vi "SetOpenWindow.vi"(8 "error in (no error)":errorcluster, 10 "Open Window":bool, 11 "object in":refnum<class "Vi_Button.lvclass">) -> (0 "error out":errorcluster, 3 "object out":refnum<class "Vi_Button.lvclass">)   [LabVIEW 2012, in "Vi_Button.lvclass"]
uses:
  Vi_Button.lvclass
  Vi_Button.lvclass/Vi_Button.ctl
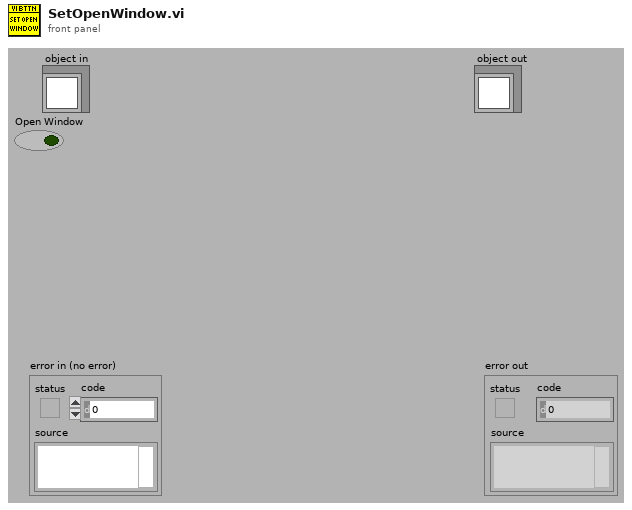
[diagram p1: front panel]
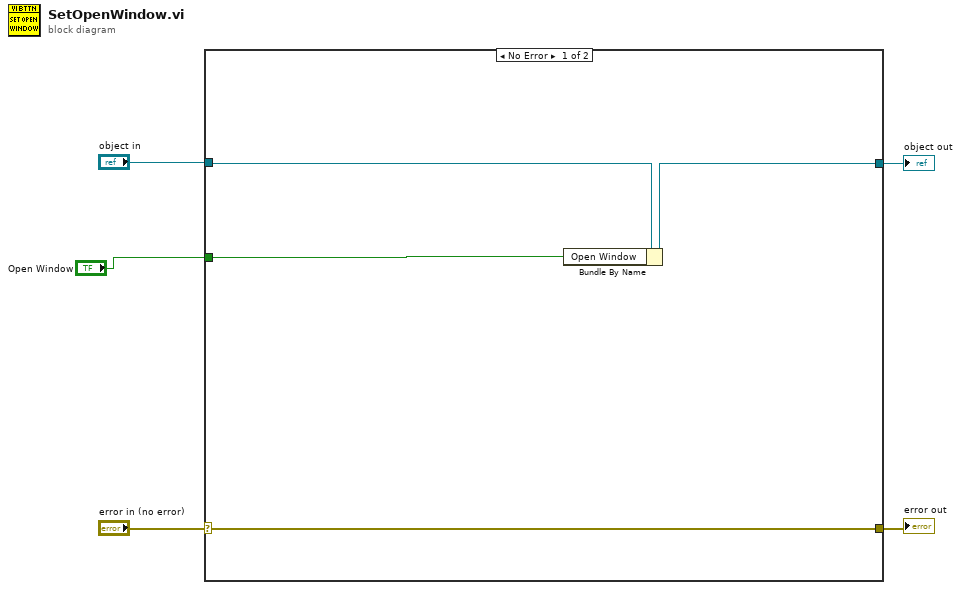
[diagram p0: block diagram]
diagram:
  n1 = case shown="No Error" "error in (no error)" {
    selector: "error in (no error)" -> [w8 w11]
    tunnel: [w8 w11] -> w4
    tunnel: [w6 w10] -> w2
    tunnel: "object in" -> [w7 w10]
    tunnel: "Open Window" -> [w9 _]
    frame No Error {
      n2 = Bundle By Name(cluster=w7, "Open Window"=w9) -> (w6:refnum<class "Vi_Button.lvclass">)
    }
    frame Error {
    }
  }
  "error out" <- w4
  "object out" <- w2
